vi "Actor Core.vi"(8 "error in":errorcluster, 11 "State in":refnum<class "Elevator.lvclass">) -> (0 "error out":errorcluster, 3 "Actor out":refnum<class "Actor.lvclass">)   [LabVIEW 2014, in "Elevator.lvlib" / "Elevator.lvclass"]
doc: "(<B>Filename</B>: Actor Framework.lvlib:Actor.lvclass:Actor Core.vi)\n\nThis override invokes Entry.vi on the initial state, prior to calling the parent Actor Core. Adding this behavior to Actor Core (instead of an override of Pre Launch Init.vi) allows the initial state to launch a nested actor as part of its entry behavior.\n\nReceives messages to the actor, reacts to them, and initiates any error handling that may shut the actor down.\n\nDescendant classes may override this VI to append parallel tasks for the actor to complete while it handles messages. Overrides use the Call Parent Method node."
uses:
  Elevator.lvclass
  <vilib>/ActorFramework/Actor/Actor.lvclass
  Elevator.lvclass/Elevator.ctl
  Motor with Encoders/Motors with Encoders Class/Motors with Encoders.lvclass
  Robot Actor Framework/System Actor/System Actor Class/System Actor.lvclass
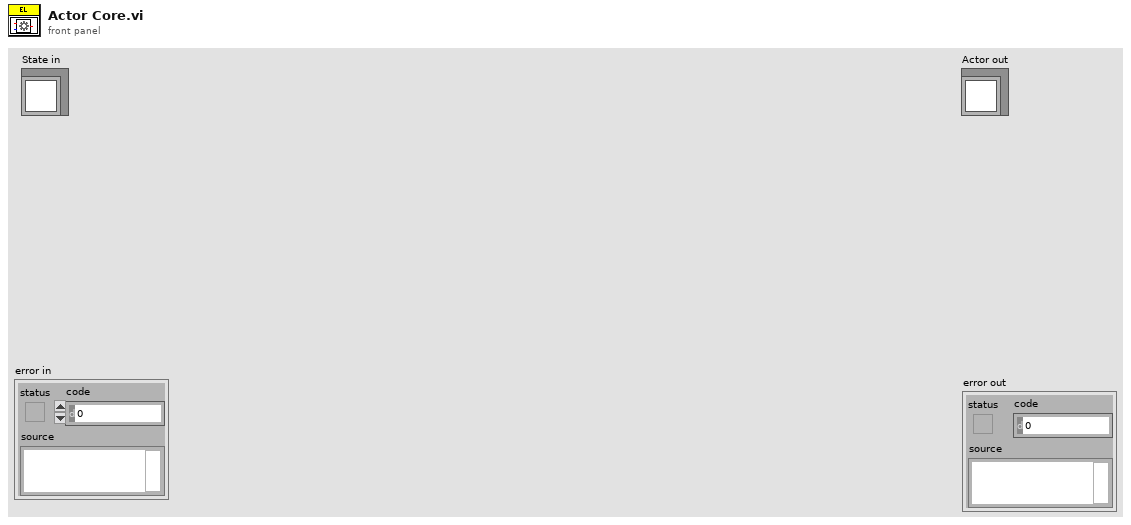
[diagram p1: front panel]
types:
  T1 = enum16{"Critical", "Error", "Warning", "Informational", "Debug"}
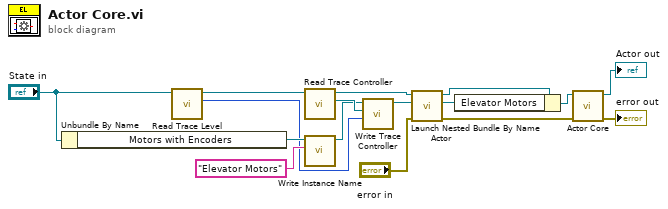
[diagram p0: block diagram]
diagram:
  n1 = Unbundle By Name("State in") -> ("Motors with Encoders"=w6:refnum<class "Motors with Encoders.lvclass">)
  n2 = call-dynamic "Read Trace Level.vi"("System Actor in"="State in") -> ("Trace Level"=w3:T1, "System Actor out"=w12:refnum<class "Elevator.lvclass">)  [unwired: 8 in, 1 out]
  n3 = call-dynamic "Read Trace Controller.vi"("System Actor in"=w12) -> ("Trace Controller"=w9:refnum<class "Message Enqueuer.lvclass">, "System Actor out"=w10:refnum<class "Elevator.lvclass">)  [unwired: 8 in, 1 out]
  n4 = call-dynamic "Write Instance Name.vi"("Instance Name"="Elevator Motors", "System Actor in"=w6) -> ("System Actor out"=w2:refnum<class "Motors with Encoders.lvclass">)  [unwired: 8 in, 1 out]
  n5 = call-dynamic "Write Trace Controller.vi"("Trace Level"=w3, "Trace Controller"=w9, "System Actor in"=w2) -> ("System Actor out"=w11:refnum<class "Motors with Encoders.lvclass">)  [unwired: 7 in, 1 out]
  n6 = call <vilib>:"Launch Nested Actor.vi"("error in (no error)"="error in", "Nested Actor"=w11, "Caller Actor in"=w10) -> ("error out"=w13:errorcluster, "Nested Actor's Enqueuer"=w5:refnum<class "Message Enqueuer.lvclass">, "Caller Actor out"=w1:refnum<class "Elevator.lvclass">)  [unwired: 6 in]
  n7 = Bundle By Name(cluster=w1, "Elevator Motors"=w5) -> (w4:refnum<class "Elevator.lvclass">)
  n8 = call-parent "Actor Core.vi"("error in"=w13, "State in"=w4) -> ("error out"=→"error out":errorcluster, "Actor out"=→"Actor out":refnum<class "Actor.lvclass">)  [unwired: 8 in]
